vi "slope.vi"() -> ()   [LabVIEW 2023]
panel:
  out "SLOPE":dbl
  in  "X1":dbl
  in  "X2":dbl
  in  "Y1":dbl
  in  "Y2":dbl
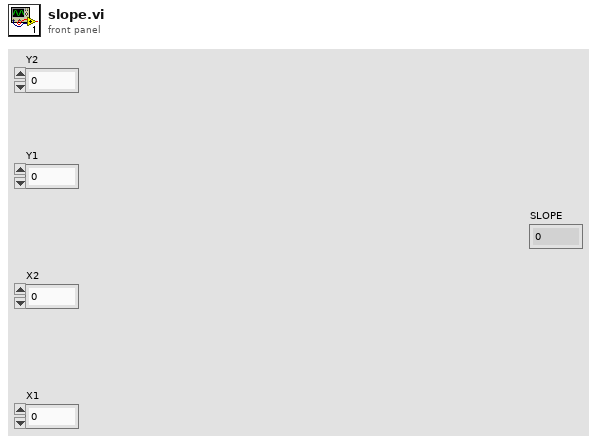
[diagram p1: front panel]
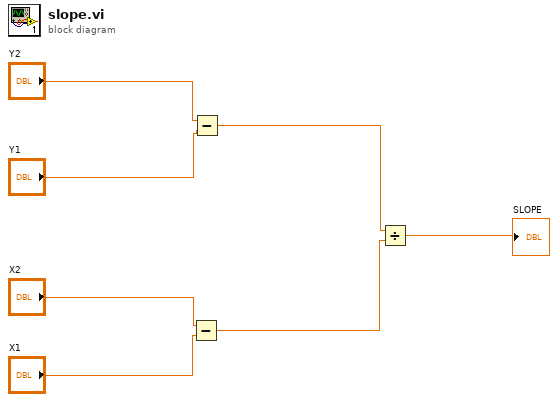
[diagram p0: block diagram]
diagram:
  n1 = Subtract(x="X2", y="X1") -> (x-y=w3:dbl)
  n2 = Subtract(x="Y2", y="Y1") -> (x-y=w2:dbl)
  n3 = Divide(x=w2, y=w3) -> (x/y=→"SLOPE":dbl)
